vi "ERR Log Error.vi"(0 "Description String":string, 11 "Error In (no error)":errorcluster) -> (10 "Logged Error String":string, 15 "Error Out":errorcluster)   [LabVIEW 2011]
doc: "This vi logs the error that has been flagge in the error.log file.\n\nThis vi was created by David Gianetto, contact me with any problems, questions, etc."
uses:
  File IO/Type Defs/FILE New Line Enum.ctl
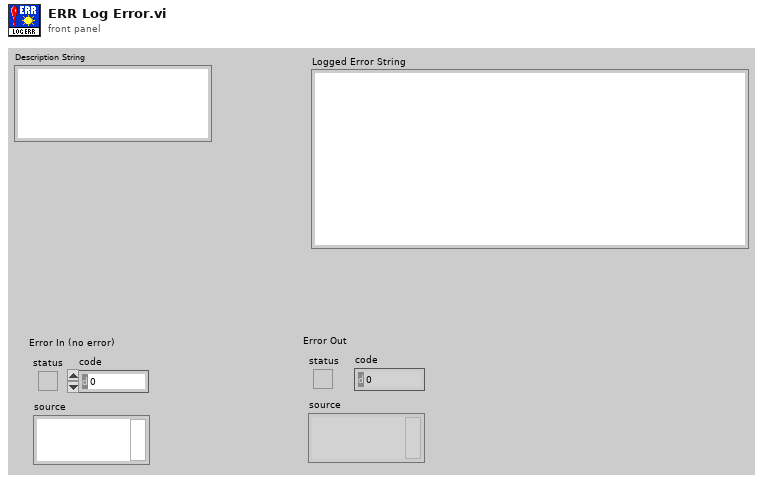
[diagram p1: front panel]
types:
  T1 = typedef "FILE New Line Enum.ctl" = enum16{"No New Line", "New Line"}
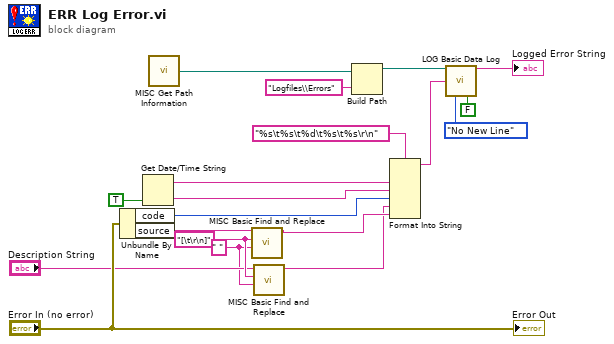
[diagram p0: block diagram]
diagram:
  w6 = " " ("Replace Text")
  w9 = "[\t\r\n]" ("Search Text")
  n1 = Unbundle By Name("Error In (no error)") -> ("code"=w17:i32, "source"=w11:string)
  n2 = Get Date/Time String(want seconds? (F)=TRUE) -> (date string=w16:string, time string=w15:string)  [unwired: 2 out]
  n3 = call "MISC Get Path Information.vi"() -> ("Support Directory"=w2:path)  [unwired: 1 in, 14 out]
  n4 = call "MISC Basic Find and Replace.vi"("Replace Text"=w6, "Search Text"=w9, "Input String"=w11) -> ("Output String"=w10:string)  [unwired: 1 in, 7 out]
  n5 = call "MISC Basic Find and Replace.vi"("Replace Text"=w6, "Search Text"=w9, "Input String"="Description String") -> ("Output String"=w7:string)  [unwired: 1 in, 7 out]
  n6 = Build Path(base path=w2, name or relative path="Logfiles\\Errors") -> (appended path=w3:path)
  n7 = Format Into String(format string="%s\t%s\t%d\t%s\t%s\r\n" ("Format String"), w16, w15, w17, w7, w10) -> (resulting string=w14:string)  [unwired: 2 in, 1 out]
  n8 = call "LOG Basic Data Log.vi"("Directory Log Path"=w3, "Line To Append"=w14, "Append Mode (new line)"=FILE_New_Line_Enum."No New Line" ("new line on append? (new line)"), "Timestamp (t:yes)"=FALSE ("Include Timestamp (t:yes)")) -> ("Logged Line"=→"Logged Error String":string)  [unwired: 3 in, 8 out]
  "Error Out" <- "Error In (no error)"
